vi "SR830_Check Time Constant and output number.vi"(8 "error in (no error)":errorcluster, 11 "SR830 resource name":refnum<visa-resource-name>) -> (0 "error out":errorcluster, 1 "TIme Constant Num":dbl, 2 "Time Constant Ring":T1(ring)=enum."300ms", 3 "SR830 resource name out":refnum<visa-resource-name>)   [LabVIEW 2019, in "User lib.lvlib"]
uses:
  User lib.lvlib
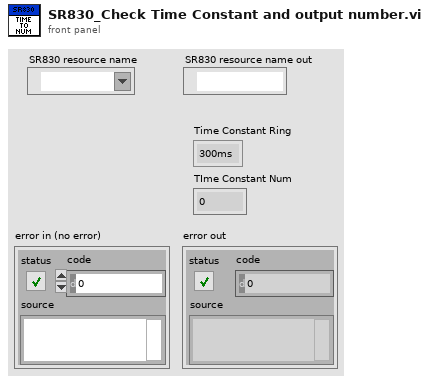
[diagram p1: front panel]
types:
  T1 = enum16{"10us", "30us", "100us", "1ms", "3ms", "5ms", "10ms", "30ms", "100ms", "300ms", "1s", "3s", "10s", "30s", "100s", "300s", "1ks", "3ks", "10ks", "30ks"}
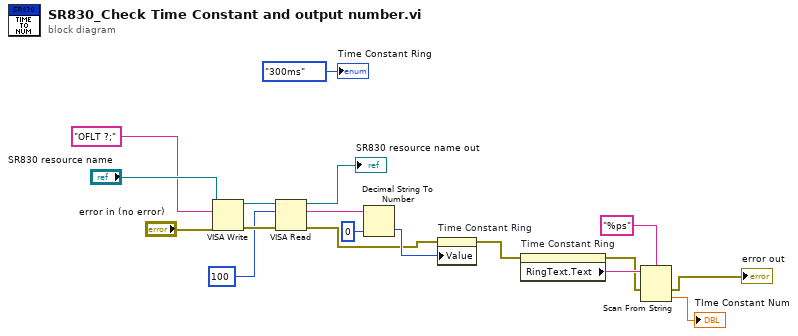
[diagram p0: block diagram]
diagram:
  n1 = VISA Write(VISA resource name="SR830 resource name", write buffer="OFLT ?;", error in (no error)="error in (no error)") -> (VISA resource name out=w13:refnum<visa-resource-name>, error out=w14:errorcluster)  [unwired: 1 out]
  n2 = VISA Read(VISA resource name=w13, byte count=u32 100, error in (no error)=w14) -> (VISA resource name out=→"SR830 resource name out":refnum<visa-resource-name>, read buffer=w11:string, error out=w8:errorcluster)  [unwired: 1 out]
  n3 = Decimal String To Number(string=w11, default (0L)=u16 0 ("default (0 I32)")) -> (number=w9:u16)  [unwired: 1 in, 1 out]
  n4 = property on="Time Constant Ring" class="Enum (strict)"(error in=w8, "Value"=w9) -> (error out=w6:errorcluster)  [unwired: 1 in, 1 out]
  n5 = property on="Time Constant Ring" class="Enum (strict)"(error in=w6) -> (error out=w4:errorcluster, "RingText.Text"=w5:string)  [unwired: 1 in, 1 out]
  n6 = Scan From String(format string="%ps", input string=w5, error in=w4) -> (error out=→"error out":errorcluster, output 1=→"TIme Constant Num":dbl)  [unwired: 2 in, 2 out]
  "Time Constant Ring" <- T1."300ms" ("Time Constant")
